vi "LEDS.vi"(10 "On/Off":bool, 11 "Type":T1) -> (0 "error out":errorcluster)   [LabVIEW 2013]
uses:
  LEDSaction.ctl
  <vilib>/Rock Robotics/SystemInterfaces/DIO/FPGA_DIOChannel.ctl
  <vilib>/Rock Robotics/SystemInterfaces/Typedef/FPGA_TypedefDigitalModule.ctl
panel:
  out "PressureHigh":bool
  out "PressureLow":bool
  out "Shoot":bool
  out "Shift":bool
  out "Hot":bool
  out "NotHot":bool
  out "10 Seconds":bool
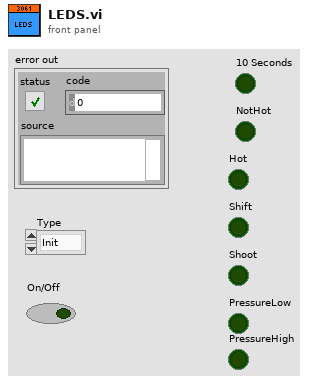
[diagram p1: front panel]
types:
  T1 = typedef "LEDSaction.ctl" = enum16{"Init", "10SecondsLeft", "LimitDown", "LimitUp", "CollectDown", "CollectUp", "NotHot", "Hot", "Shift", "RollBack", "RollFwd", "Shoot", "Distance Low", "DistanceHigh", "PressureLow", "PressureHigh"}
  T2 = typedef "FPGA_DIOChannel.ctl" = enum8{"DIO 1", "DIO 2", "DIO 3", "DIO 4", "DIO 5", "DIO 6", "DIO 7", "DIO 8", "DIO 9", "DIO 10", "DIO 11", "DIO 12", "DIO 13", "DIO 14", "Invalid"}
  T3 = typedef "FPGA_TypedefDigitalModule.ctl" = enum16{"Digital Module 1", "Digital Module 2"}
  T4 = typedef "WPI_DigitalOutputDevRef.ctl" = cluster{"Digital Module":T3, "DIO Channel":T2, "DevStatus":errorcluster}
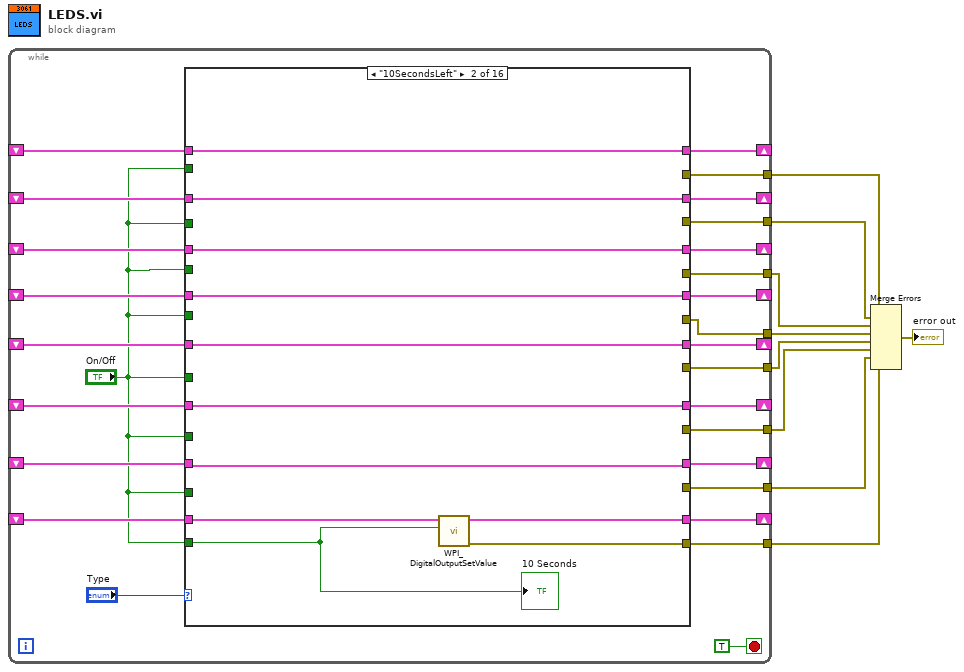
[diagram p0: block diagram]
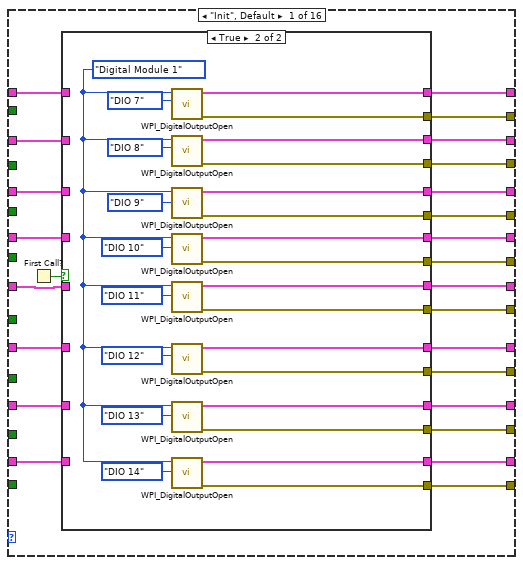
[diagram p2: hidden frame]
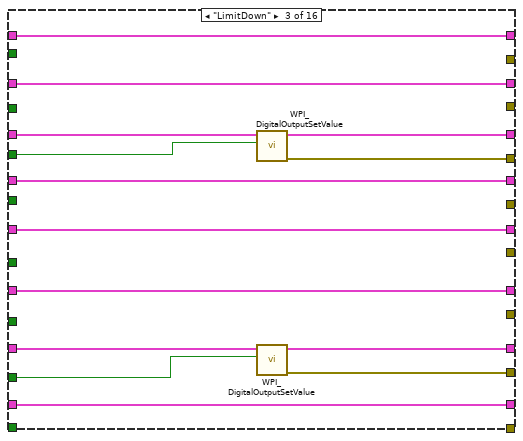
[diagram p4: hidden frame]
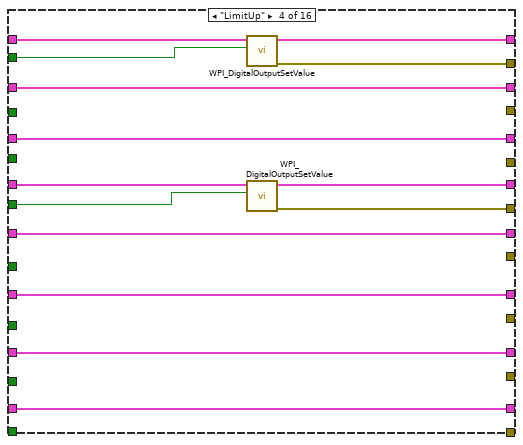
[diagram p5: hidden frame]
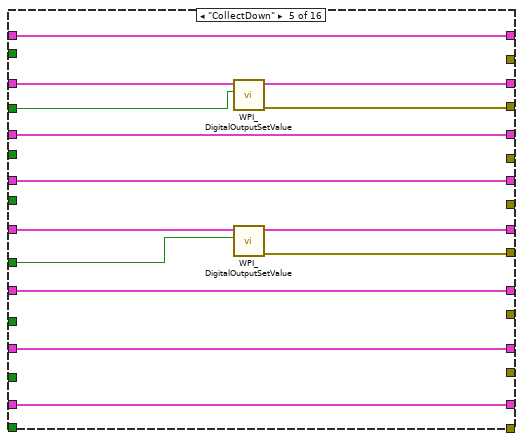
[diagram p6: hidden frame]
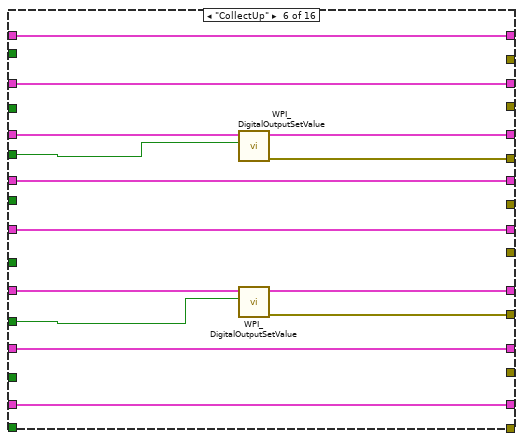
[diagram p7: hidden frame]
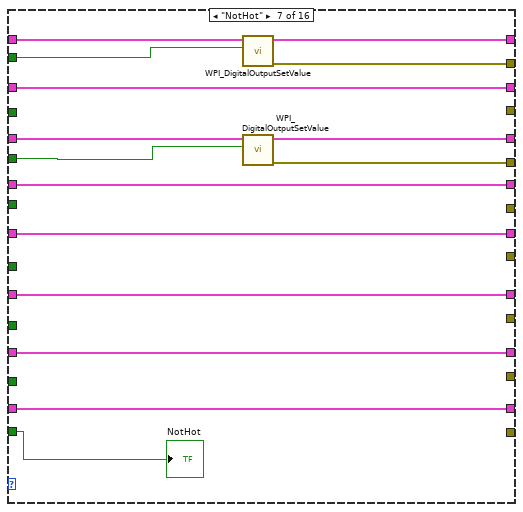
[diagram p8: hidden frame]
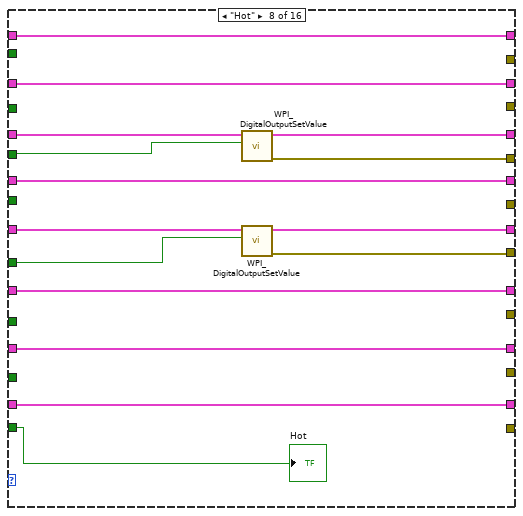
[diagram p9: hidden frame]
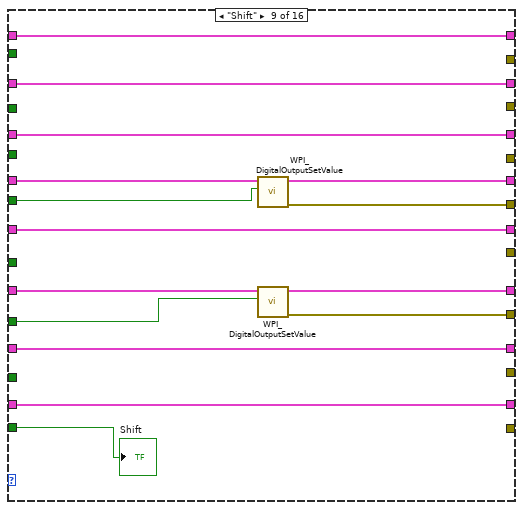
[diagram p10: hidden frame]
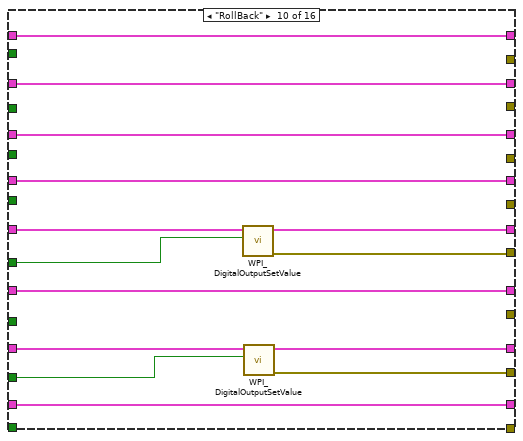
[diagram p11: hidden frame]
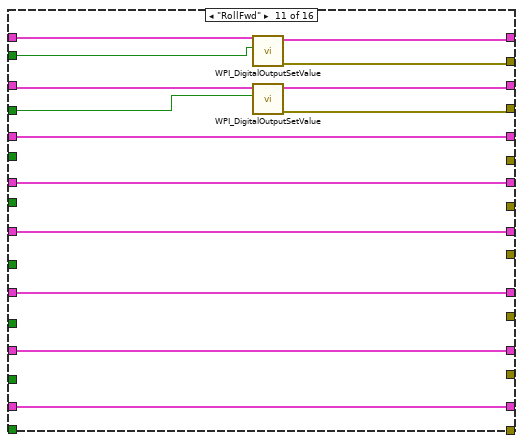
[diagram p12: hidden frame]
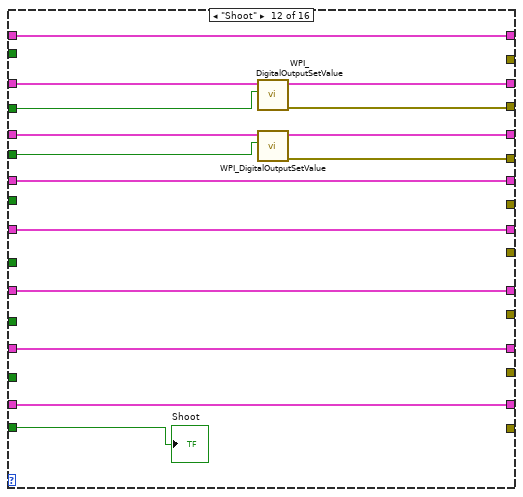
[diagram p13: hidden frame]
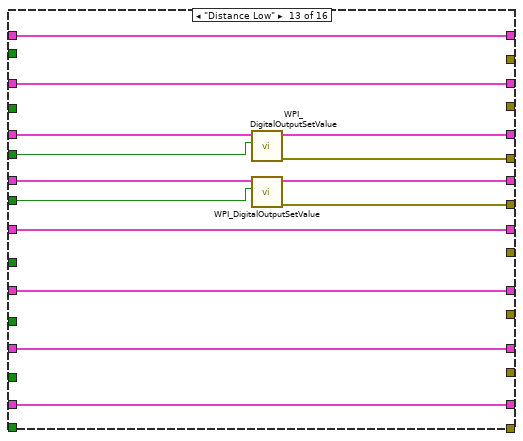
[diagram p14: hidden frame]
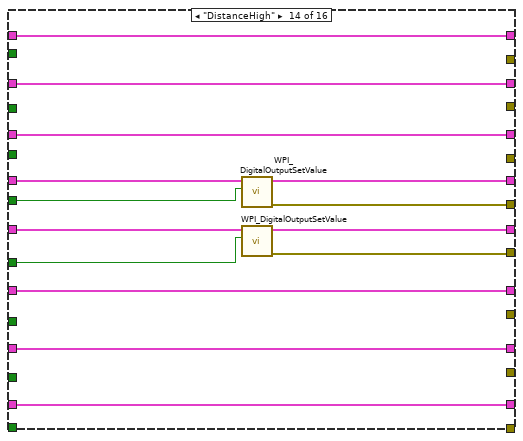
[diagram p15: hidden frame]
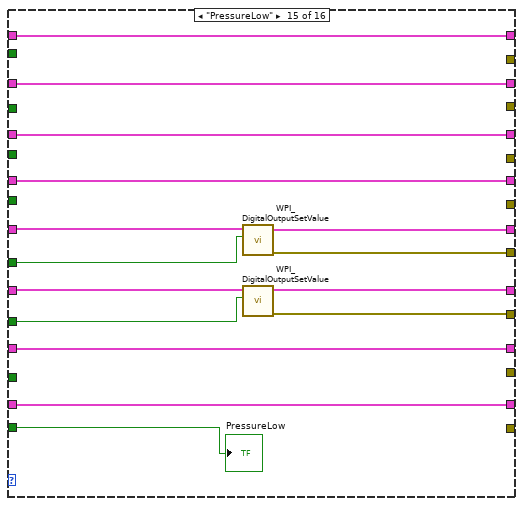
[diagram p16: hidden frame]
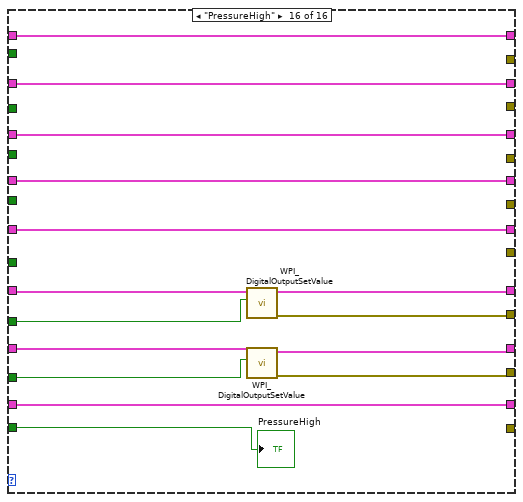
[diagram p17: hidden frame]
diagram:
  n1 = while {
    shift-right: [w36] -> _
    shift-left: _ -> [w28]
    shift-right: [w35] -> _
    shift-left: _ -> [w27]
    shift-right: [w34] -> _
    shift-left: _ -> [w26]
    shift-right: [w33] -> _
    shift-left: _ -> [w25]
    shift-right: [w32] -> _
    shift-left: _ -> [w24]
    shift-right: [w31] -> _
    shift-left: _ -> [w23]
    shift-right: [w30] -> _
    shift-left: _ -> [w22]
    shift-right: [w29] -> _
    shift-left: _ -> [w21]
    tunnel: [w19] -> w8
    tunnel: [w18] -> w7
    tunnel: [w17] -> w6
    tunnel: [w16] -> w5
    tunnel: [w15] -> w4
    tunnel: [w14] -> w3
    tunnel: [w13] -> w2
    tunnel: [w12] -> w1
    stop <- TRUE stop-if-true
    n2 = case shown="\"10SecondsLeft\"" "Type" {
      tunnel: [w46 w103 w110 w133 w143 w157 w175 w185 w199 w211 w234 w245 w259 w271 w283 w298] -> w36
      tunnel: [w48 w102 w111 w128 w147 w156 w172 w186 w200 w212 w233 w249 w258 w272 w284 w299] -> w35
      tunnel: [w50 w101 w118 w129 w142 w161 w176 w191 w201 w213 w230 w248 w263 w273 w285 w300] -> w34
      tunnel: [w52 w100 w112 w132 w141 w155 w171 w187 w205 w214 w229 w244 w262 w276 w286 w301] -> w33
      tunnel: [w54 w99 w113 w127 w146 w154 w170 w190 w202 w219 w228 w243 w257 w277 w291 w302] -> w32
      tunnel: [w56 w98 w114 w126 w140 w160 w169 w184 w206 w216 w227 w242 w256 w270 w292 w306] -> w31
      tunnel: [w58 w97 w117 w125 w139 w153 w168 w183 w198 w220 w226 w241 w255 w269 w288 w307] -> w30
      tunnel: [w60 w104 w115 w124 w138 w152 w167 w182 w197 w215 w225 w240 w254 w268 w287 w303] -> w29
      tunnel: w28 -> [w37 w103 w110 w131 w143 w157 w174 w185 w199 w211 w231 w245 w259 w271 w283 w298]
      tunnel: w27 -> [w38 w102 w111 w128 w144 w156 w172 w186 w200 w212 w232 w246 w258 w272 w284 w299]
      tunnel: w26 -> [w39 w101 w119 w129 w142 w158 w173 w189 w201 w213 w230 w247 w260 w273 w285 w300]
      tunnel: w25 -> [w40 w100 w112 w130 w141 w155 w171 w187 w204 w214 w229 w244 w261 w275 w286 w301]
      tunnel: w24 -> [w44 w99 w113 w127 w145 w154 w170 w188 w202 w217 w228 w243 w257 w274 w290 w302]
      tunnel: w23 -> [w43 w98 w114 w126 w140 w159 w169 w184 w203 w216 w227 w242 w256 w270 w289 w305]
      tunnel: w22 -> [w42 w97 w116 w125 w139 w153 w168 w183 w198 w218 w226 w241 w255 w269 w288 w304]
      tunnel: w21 -> [w41 w105 w115 w124 w138 w152 w167 w182 w197 w215 w225 w240 w254 w268 w287 w303]
      tunnel: [w47 _ _ w123 _ _ w166 _ _ _ w224 _ _ _ _ _] -> w12
      tunnel: [w49 _ _ _ w137 _ _ _ _ _ w223 w239 _ _ _ _] -> w13
      tunnel: [w51 _ w109 _ _ w151 w165 w181 _ _ _ w238 w253 _ _ _] -> w14
      tunnel: [w53 _ _ w122 _ _ _ _ w196 _ _ _ w252 w267 _ _] -> w15
      tunnel: [w55 _ _ _ w136 _ _ w180 _ w210 _ _ _ w266 w282 _] -> w16
      tunnel: [w57 _ _ _ _ w150 _ _ w195 _ _ _ _ _ w281 w297] -> w17
      tunnel: [w59 _ w108 _ _ _ _ _ _ w209 _ _ _ _ _ w296] -> w18
      tunnel: [w61 w96 _ _ _ _ _ _ _ _ _ _ _ _ _ _] -> w19
      tunnel: "On/Off" -> [_ _ _ _ w134 _ _ w178 _ w208 _ _ _ w264 w280 _]
      tunnel: "On/Off" -> [_ _ _ w121 _ _ w164 _ _ _ w221 _ _ _ _ _]
      tunnel: "On/Off" -> [_ _ _ _ w135 _ _ _ _ _ w222 w237 _ _ _ _]
      tunnel: "On/Off" -> [_ _ w106 _ _ w149 w163 w179 _ _ _ w236 w251 _ _ _]
      tunnel: "On/Off" -> [_ _ _ w120 _ _ _ _ w194 _ _ _ w250 w265 _ _]
      tunnel: "On/Off" -> [_ w95 _ _ _ _ w162 w177 w192 _ _ w235 _ _ w278 w293]
      tunnel: "On/Off" -> [_ _ w107 _ _ _ _ _ _ w207 _ _ _ _ _ w294]
      tunnel: "On/Off" -> [_ _ _ _ _ w148 _ _ w193 _ _ _ _ _ w279 w295]
      frame "Init", Default {
        n3 = First Call?() -> (First Call?: T/F=w45:bool)
        n4 = case shown="True" w45 {
          tunnel: [_ w86] -> w61
          tunnel: [w66 w85] -> w60
          tunnel: [_ w84] -> w59
          tunnel: [w67 w83] -> w58
          tunnel: [_ w82] -> w57
          tunnel: [w68 w81] -> w56
          tunnel: [_ w80] -> w55
          tunnel: [w69 w79] -> w54
          tunnel: [_ w78] -> w53
          tunnel: [w65 w77] -> w52
          tunnel: [_ w76] -> w51
          tunnel: [w64 w75] -> w50
          tunnel: [_ w74] -> w49
          tunnel: [w63 w73] -> w48
          tunnel: [_ w72] -> w47
          tunnel: [w62 w71] -> w46
          tunnel: w44 -> [w69 _]
          tunnel: w43 -> [w68 _]
          tunnel: w42 -> [w67 _]
          tunnel: w41 -> [w66 _]
          tunnel: w40 -> [w65 _]
          tunnel: w39 -> [w64 _]
          tunnel: w38 -> [w63 _]
          tunnel: w37 -> [w62 _]
          frame False {
          }
          frame True {
            w70 = FPGA_TypedefDigitalModule."Digital Module 1" ("Digital Module (Module 1)")
            n5 = call <vilib>:"WPI_DigitalOutputOpen.vi"("DIO Channel"=FPGA_DIOChannel."DIO 7", "Digital Module (Module 1)"=w70) -> ("error out"=w72:errorcluster, "DigitalOutputDevRef"=w71:T4)  [unwired: 8 in]
            n6 = call <vilib>:"WPI_DigitalOutputOpen.vi"("DIO Channel"=FPGA_DIOChannel."DIO 8", "Digital Module (Module 1)"=w70) -> ("error out"=w74:errorcluster, "DigitalOutputDevRef"=w73:T4)  [unwired: 8 in]
            n7 = call <vilib>:"WPI_DigitalOutputOpen.vi"("DIO Channel"=FPGA_DIOChannel."DIO 9", "Digital Module (Module 1)"=w70) -> ("error out"=w76:errorcluster, "DigitalOutputDevRef"=w75:T4)  [unwired: 8 in]
            n8 = call <vilib>:"WPI_DigitalOutputOpen.vi"("DIO Channel"=FPGA_DIOChannel."DIO 10", "Digital Module (Module 1)"=w70) -> ("error out"=w78:errorcluster, "DigitalOutputDevRef"=w77:T4)  [unwired: 8 in]
            n9 = call <vilib>:"WPI_DigitalOutputOpen.vi"("DIO Channel"=FPGA_DIOChannel."DIO 11", "Digital Module (Module 1)"=w70) -> ("error out"=w80:errorcluster, "DigitalOutputDevRef"=w79:T4)  [unwired: 8 in]
            n10 = call <vilib>:"WPI_DigitalOutputOpen.vi"("DIO Channel"=FPGA_DIOChannel."DIO 12", "Digital Module (Module 1)"=w70) -> ("error out"=w82:errorcluster, "DigitalOutputDevRef"=w81:T4)  [unwired: 8 in]
            n11 = call <vilib>:"WPI_DigitalOutputOpen.vi"("DIO Channel"=FPGA_DIOChannel."DIO 13", "Digital Module (Module 1)"=w70) -> ("error out"=w84:errorcluster, "DigitalOutputDevRef"=w83:T4)  [unwired: 8 in]
            n12 = call <vilib>:"WPI_DigitalOutputOpen.vi"("DIO Channel"=FPGA_DIOChannel."DIO 14", "Digital Module (Module 1)"=w70) -> ("error out"=w86:errorcluster, "DigitalOutputDevRef"=w85:T4)  [unwired: 8 in]
          }
        }
      }
      frame "10SecondsLeft" {
        n13 = call <vilib>:"WPI_DigitalOutputSetValue.vi"("Value"=w95, "DigitalOutputDevRef"=w105) -> ("error out"=w96:errorcluster, "DigitalOutputDevRef"=w104:T4)  [unwired: 8 in]
        "10 Seconds" <- w95
      }
      frame "LimitDown" {
        n14 = call <vilib>:"WPI_DigitalOutputSetValue.vi"("Value"=w106, "DigitalOutputDevRef"=w119) -> ("error out"=w109:errorcluster, "DigitalOutputDevRef"=w118:T4)  [unwired: 8 in]
        n15 = call <vilib>:"WPI_DigitalOutputSetValue.vi"("Value"=w107, "DigitalOutputDevRef"=w116) -> ("error out"=w108:errorcluster, "DigitalOutputDevRef"=w117:T4)  [unwired: 8 in]
      }
      frame "LimitUp" {
        n16 = call <vilib>:"WPI_DigitalOutputSetValue.vi"("Value"=w121, "DigitalOutputDevRef"=w131) -> ("error out"=w123:errorcluster, "DigitalOutputDevRef"=w133:T4)  [unwired: 8 in]
        n17 = call <vilib>:"WPI_DigitalOutputSetValue.vi"("Value"=w120, "DigitalOutputDevRef"=w130) -> ("error out"=w122:errorcluster, "DigitalOutputDevRef"=w132:T4)  [unwired: 8 in]
      }
      frame "CollectDown" {
        n18 = call <vilib>:"WPI_DigitalOutputSetValue.vi"("Value"=w135, "DigitalOutputDevRef"=w144) -> ("error out"=w137:errorcluster, "DigitalOutputDevRef"=w147:T4)  [unwired: 8 in]
        n19 = call <vilib>:"WPI_DigitalOutputSetValue.vi"("Value"=w134, "DigitalOutputDevRef"=w145) -> ("error out"=w136:errorcluster, "DigitalOutputDevRef"=w146:T4)  [unwired: 8 in]
      }
      frame "CollectUp" {
        n20 = call <vilib>:"WPI_DigitalOutputSetValue.vi"("Value"=w149, "DigitalOutputDevRef"=w158) -> ("error out"=w151:errorcluster, "DigitalOutputDevRef"=w161:T4)  [unwired: 8 in]
        n21 = call <vilib>:"WPI_DigitalOutputSetValue.vi"("Value"=w148, "DigitalOutputDevRef"=w159) -> ("error out"=w150:errorcluster, "DigitalOutputDevRef"=w160:T4)  [unwired: 8 in]
      }
      frame "NotHot" {
        n22 = call <vilib>:"WPI_DigitalOutputSetValue.vi"("Value"=w164, "DigitalOutputDevRef"=w174) -> ("error out"=w166:errorcluster, "DigitalOutputDevRef"=w175:T4)  [unwired: 8 in]
        n23 = call <vilib>:"WPI_DigitalOutputSetValue.vi"("Value"=w163, "DigitalOutputDevRef"=w173) -> ("error out"=w165:errorcluster, "DigitalOutputDevRef"=w176:T4)  [unwired: 8 in]
        "NotHot" <- w162
      }
      frame "Hot" {
        n24 = call <vilib>:"WPI_DigitalOutputSetValue.vi"("Value"=w179, "DigitalOutputDevRef"=w189) -> ("error out"=w181:errorcluster, "DigitalOutputDevRef"=w191:T4)  [unwired: 8 in]
        n25 = call <vilib>:"WPI_DigitalOutputSetValue.vi"("Value"=w178, "DigitalOutputDevRef"=w188) -> ("error out"=w180:errorcluster, "DigitalOutputDevRef"=w190:T4)  [unwired: 8 in]
        "Hot" <- w177
      }
      frame "Shift" {
        n26 = call <vilib>:"WPI_DigitalOutputSetValue.vi"("Value"=w194, "DigitalOutputDevRef"=w204) -> ("error out"=w196:errorcluster, "DigitalOutputDevRef"=w205:T4)  [unwired: 8 in]
        n27 = call <vilib>:"WPI_DigitalOutputSetValue.vi"("Value"=w193, "DigitalOutputDevRef"=w203) -> ("error out"=w195:errorcluster, "DigitalOutputDevRef"=w206:T4)  [unwired: 8 in]
        "Shift" <- w192
      }
      frame "RollBack" {
        n28 = call <vilib>:"WPI_DigitalOutputSetValue.vi"("Value"=w208, "DigitalOutputDevRef"=w217) -> ("error out"=w210:errorcluster, "DigitalOutputDevRef"=w219:T4)  [unwired: 8 in]
        n29 = call <vilib>:"WPI_DigitalOutputSetValue.vi"("Value"=w207, "DigitalOutputDevRef"=w218) -> ("error out"=w209:errorcluster, "DigitalOutputDevRef"=w220:T4)  [unwired: 8 in]
      }
      frame "RollFwd" {
        n30 = call <vilib>:"WPI_DigitalOutputSetValue.vi"("Value"=w221, "DigitalOutputDevRef"=w231) -> ("error out"=w224:errorcluster, "DigitalOutputDevRef"=w234:T4)  [unwired: 8 in]
        n31 = call <vilib>:"WPI_DigitalOutputSetValue.vi"("Value"=w222, "DigitalOutputDevRef"=w232) -> ("error out"=w223:errorcluster, "DigitalOutputDevRef"=w233:T4)  [unwired: 8 in]
      }
      frame "Shoot" {
        n32 = call <vilib>:"WPI_DigitalOutputSetValue.vi"("Value"=w237, "DigitalOutputDevRef"=w246) -> ("error out"=w239:errorcluster, "DigitalOutputDevRef"=w249:T4)  [unwired: 8 in]
        n33 = call <vilib>:"WPI_DigitalOutputSetValue.vi"("Value"=w236, "DigitalOutputDevRef"=w247) -> ("error out"=w238:errorcluster, "DigitalOutputDevRef"=w248:T4)  [unwired: 8 in]
        "Shoot" <- w235
      }
      frame "Distance Low" {
        n34 = call <vilib>:"WPI_DigitalOutputSetValue.vi"("Value"=w251, "DigitalOutputDevRef"=w260) -> ("error out"=w253:errorcluster, "DigitalOutputDevRef"=w263:T4)  [unwired: 8 in]
        n35 = call <vilib>:"WPI_DigitalOutputSetValue.vi"("Value"=w250, "DigitalOutputDevRef"=w261) -> ("error out"=w252:errorcluster, "DigitalOutputDevRef"=w262:T4)  [unwired: 8 in]
      }
      frame "DistanceHigh" {
        n36 = call <vilib>:"WPI_DigitalOutputSetValue.vi"("Value"=w265, "DigitalOutputDevRef"=w275) -> ("error out"=w267:errorcluster, "DigitalOutputDevRef"=w276:T4)  [unwired: 8 in]
        n37 = call <vilib>:"WPI_DigitalOutputSetValue.vi"("Value"=w264, "DigitalOutputDevRef"=w274) -> ("error out"=w266:errorcluster, "DigitalOutputDevRef"=w277:T4)  [unwired: 8 in]
      }
      frame "PressureLow" {
        n38 = call <vilib>:"WPI_DigitalOutputSetValue.vi"("Value"=w280, "DigitalOutputDevRef"=w290) -> ("error out"=w282:errorcluster, "DigitalOutputDevRef"=w291:T4)  [unwired: 8 in]
        n39 = call <vilib>:"WPI_DigitalOutputSetValue.vi"("Value"=w279, "DigitalOutputDevRef"=w289) -> ("error out"=w281:errorcluster, "DigitalOutputDevRef"=w292:T4)  [unwired: 8 in]
        "PressureLow" <- w278
      }
      frame "PressureHigh" {
        n40 = call <vilib>:"WPI_DigitalOutputSetValue.vi"("Value"=w295, "DigitalOutputDevRef"=w305) -> ("error out"=w297:errorcluster, "DigitalOutputDevRef"=w306:T4)  [unwired: 8 in]
        n41 = call <vilib>:"WPI_DigitalOutputSetValue.vi"("Value"=w294, "DigitalOutputDevRef"=w304) -> ("error out"=w296:errorcluster, "DigitalOutputDevRef"=w307:T4)  [unwired: 8 in]
        "PressureHigh" <- w293
      }
    }
  }
  n42 = Merge Errors(w1, w2, w3, w4, w5, w6, w7, w8) -> (→"error out":errorcluster)
